vi "Example1.vi"() -> ()   [LabVIEW 2020]
doc: "Basic example of advantage type definitions."
uses:
  Ctrl/PointCluster.ctl
panel:
  in  "Tab":enum32{"Normal", "Typedef"}(tab)
  in  "Cluster1":T1 caption="Example Cluster 1"
  in  "x":dbl
  in  "y":dbl
  in  "z":dbl
  in  "Description":string
  out "Out":T1
  in  "x 2":dbl
  in  "y 2":dbl
  in  "z 2":dbl
  in  "Description 2":string
  in  "Cluster2":T2 caption="Example Cluster 2"
  out "Out 2":T2 caption="Out"
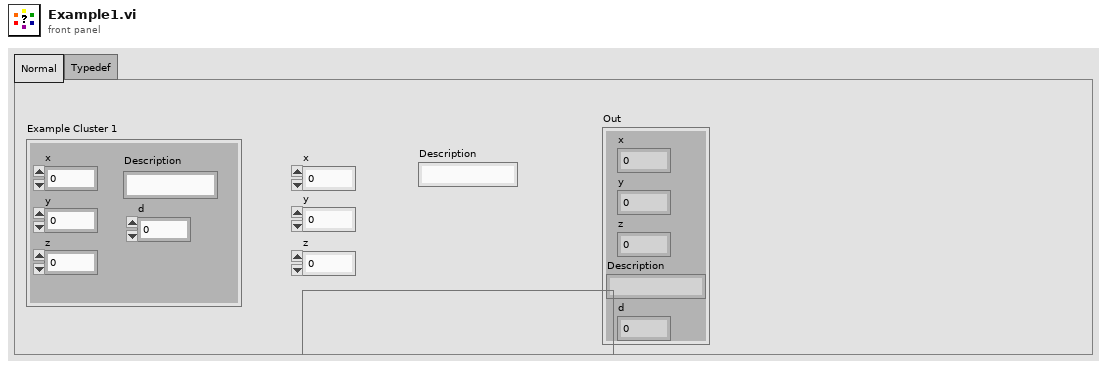
[diagram p1: front panel]
types:
  T1 = cluster{"x":dbl, "y":dbl, "z ":dbl, "Description":string, "d":dbl}
  T2 = typedef "PointCluster.ctl" = cluster{"x":dbl, "y":dbl, "z ":dbl, "Description":string, "d":dbl}
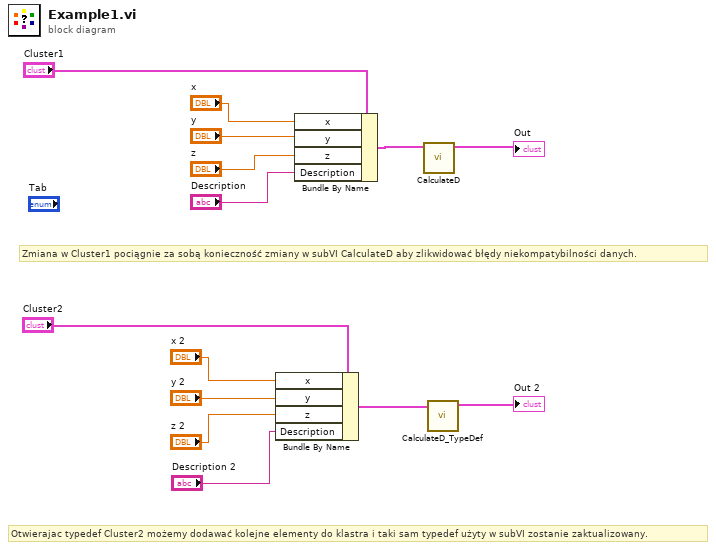
[diagram p0: block diagram]
diagram:
  # "Otwierajac typedef Cluster2 możemy dodawać kolejne elementy do klastra i taki sam typedef użyty w subVI zostanie zaktualizowany."
  # "Zmiana w Cluster1 pociągnie za sobą konieczność zmiany w subVI CalculateD aby zlikwidować błędy niekompatybilności danych."
  n1 = Bundle By Name(cluster="Cluster2", "x"="x 2", "y"="y 2", "z"="z 2", "Description"="Description 2") -> (w3:T2)
  n2 = Bundle By Name(cluster="Cluster1", "x"="x", "y"="y", "z"="z", "Description"="Description") -> (w10:T1)
  n3 = call "CalculateD.vi"("Cluster In"=w10) -> ("Cluster Out"=→"Out":T1)  [unwired: 10 in]
  n4 = call "CalculateD_TypeDef.vi"("Cluster In"=w3) -> ("output cluster"=→"Out 2":T2)  [unwired: 10 in]
